vi "bug exec init.vi"() -> (8 "exp exec":T2={"data file"={"autosave"=FALSE, "File refnum"=refnum, "data file path"=path ""}, "T log file"={"File refnum"=refnum, "T log file path"=path "", "exists"=FALSE}, "exp seq"={"wave params"={"Num of avg"=0, "Num points"=0, "Meas rate (Hz)"=0.0}, "Setpoints"=[], "#"=0, "index"=0, "elapsed time (s)"=0.0, "set time (s)"=0.0, "min settle (s)"=30.0, " Exec Status"=enum."Settling"}, "error"={"status"=FALSE, "code"=0, "source"=""}})   [LabVIEW 2019]
doc: "This is a Bug C(T) subVI.\n\nIt initializes the exec cluster for proper operation.\n\nPaul K Dixon\nP3600\nCSUSB Physics"
uses:
  typedefs/PID exec cluster.ctl
  typedefs/data file info.ctl
  typedefs/bug temp file info.ctl
  typedefs/exp seq cluster.ctl
  typedefs/wvfm acq params.ctl
  typedefs/bug meas status.ctl
panel:
  in  "wave params":T1={"Num of avg"=10, "Num points"=1000, "Meas rate (Hz)"=100000.0}
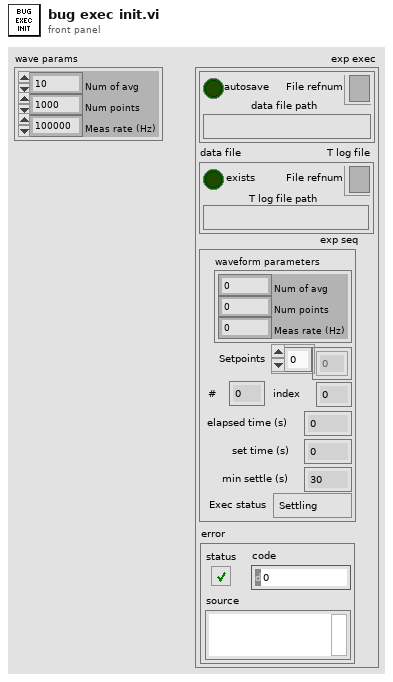
[diagram p1: front panel]
types:
  T1 = typedef "wvfm acq params.ctl" = cluster{"Num of avg":i32, "Num points":i32, "Meas rate (Hz)":dbl}
  T2 = typedef "PID exec cluster.ctl" = cluster{"data file":T3, "T log file":T4, "exp seq":T5, "error":errorcluster}
  T3 = typedef "data file info.ctl" = cluster{"autosave":bool, "File refnum":refnum<file>, "data file path":path}
  T4 = typedef "bug temp file info.ctl" = cluster{"File refnum":refnum<file>, "T log file path":path, "exists":bool}
  T5 = typedef "exp seq cluster.ctl" = cluster{"wave params":T1, "Setpoints":dbl[], "#":i32, "index":i32, "elapsed time (s)":dbl, "set time (s)":dbl, "min settle (s)":dbl, " Exec Status":T6}
  T6 = typedef "bug meas status.ctl" = enum32{"Settling", "Measuring", "Holding", "Exit"}
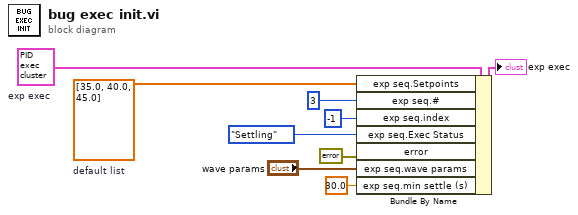
[diagram p0: block diagram]
diagram:
  w7 = dbl[] [35.0, 40.0, 45.0]  # default list
  w8 = T2 {"data file"={"autosave"=FALSE, "File refnum"=refnum, "data file path"=path ""}, "T log file"={"File refnum"=refnum, "T log file path"=path "", "exists"=FALSE}, "exp seq"={"wave params"={"Num of avg"=0, "Num points"=0, "Meas rate (Hz)"=0.0}, "Setpoints"=[], "#"=0, "index"=0, "elapsed time (s)"=0.0, "set time (s)"=0.0, "min settle (s)"=30.0, " Exec Status"=enum."Settling"}, "error"={"status"=FALSE, "code"=0, "source"=""}}  # exp exec
  n1 = Bundle By Name(cluster=w8, "exp seq.Setpoints"=w7, "exp seq.#"=3, "exp seq.index"=-1, "exp seq.Exec Status"=bug_meas_status."Settling" ("exp seq. Exec Status"), "error"=errorcluster {"status"=FALSE, "code"=0, "source"=""}, "exp seq.wave params"="wave params", "exp seq.min settle (s)"=30.0) -> (→"exp exec":T2)
